vi "FTW-Inbox-Core-ConstructMessagePipe.vi"(5 "Actor Identity (empty to create unnamed actor)":string, 7 "Is Primary?":bool=TRUE, 11 "error in":errorcluster) -> (4 "Message Pipe":refnum<queue>, 6 "Resolved Actor Identity":string, 15 "error out":errorcluster)   [LabVIEW 2015]
uses:
  core/type/FTW-Type-JSON.ctl
panel:
  # "Inputs"
  # "Outputs"
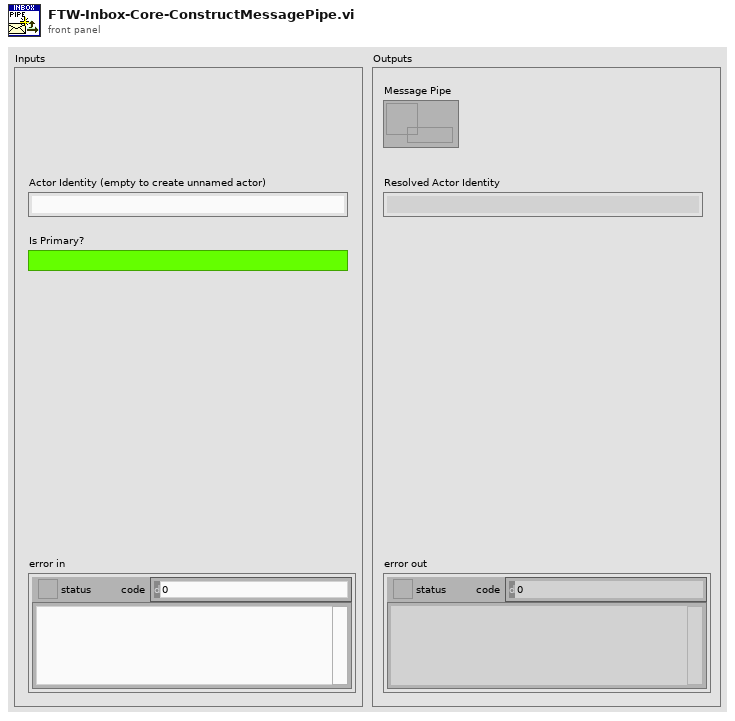
[diagram p1: front panel]
types:
  T1 = typedef "FTW-Type-JSON.ctl" = refnum<data-value>
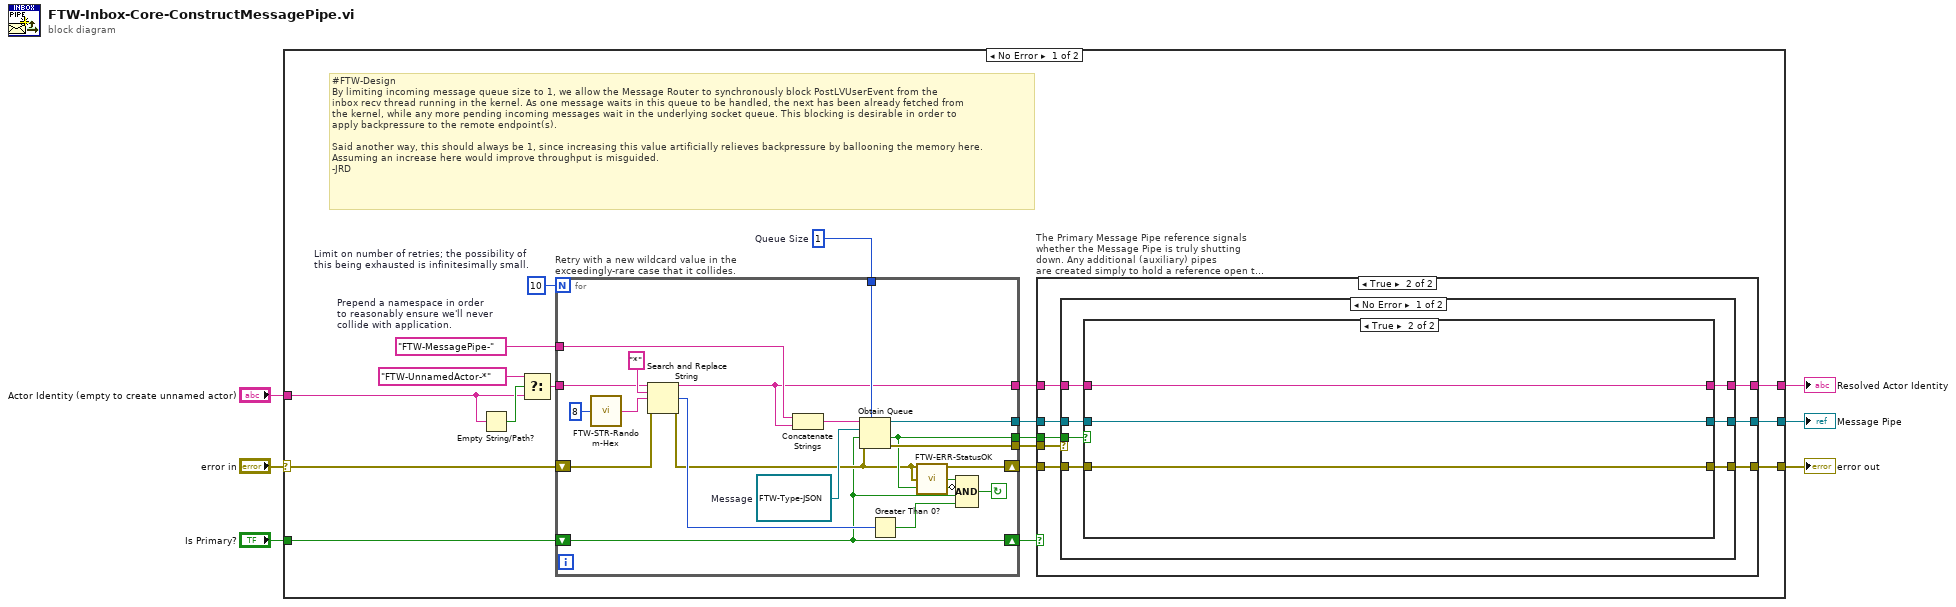
[diagram p0: block diagram]
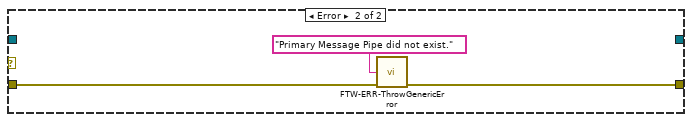
[diagram p3: hidden frame]
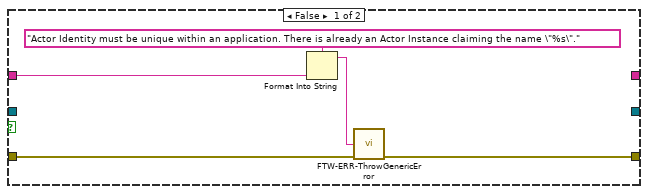
[diagram p4: hidden frame]
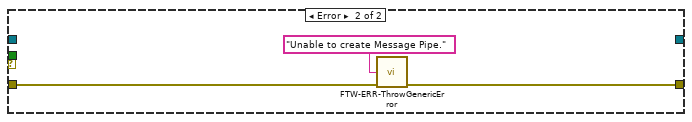
[diagram p5: hidden frame]
diagram:
  n1 = case shown="No Error" "error in" {
    selector: "error in" -> [w14 w83]
    tunnel: [w23 _] -> w6
    tunnel: "Actor Identity (empty to create unnamed actor)" -> [w16 _]
    tunnel: "Is Primary?" -> [w18 _]
    tunnel: [w24 w83] -> w3
    tunnel: [w19 _] -> w1
    frame No Error {
      w7 = "FTW-MessagePipe-"  # Prepend a namespace in order to reasonably ensure we'll never collide with application.
      w10 = 1  # Queue Size
      w11 = 10  # Limit on number of retries; the possibility of this being exhausted is infinitesimally small.
      # "#FTW-Design\nBy limiting incoming message queue size to 1, we allow the Message Router to synchronously block PostLVUserEvent from the\ninbox recv thread running in the kernel. As one message waits in this queue to be handled, the next has been already fetched from\nthe kernel, while any more pending incoming messages wait in the underlying socket queue. This blocking is desirable in order to\napply backpressure to the remote endpoint(s).\n\nSaid another way, this should always be 1, since increasing this value artificially relieves backpressure by ballooning the memory here.\nAssuming an increase here would improve throughput is misguided.\n-JRD"
      n2 = Empty String/Path?(string/path=w16) -> (empty?=w17:bool)
      n3 = Select(t="FTW-UnnamedActor-*" ("string"), s=w17, f=w16) -> (s? t:f=w8:string)
      n4 = for "Retry with a new wildcard value in the exceedingly-rare case that it collides." {
        N: w11 -> [_]
        tunnel: [w42] -> w21
        tunnel: [w41] -> w20
        shift-right: [w32] -> w13
        shift-left: w14 -> [w37]
        tunnel: [w33] -> w22
        tunnel: w8 -> [w34]
        tunnel: [w26] -> w12
        tunnel: w10 -> [w29]
        shift-right: [w28] -> w9
        shift-left: w18 -> [w28]
        tunnel: w7 -> [w27]
        stop <- w30 continue-if-true
        w43 = T1 refnum  # Message
        n5 = call "FTW-STR-Random-Hex.vi"("String Length"=8) -> ("Random Hex String"=w40:string)  [unwired: 3 in]
        n6 = Search and Replace String(input string=w34, search string="*", replace string=w40, error in=w37) -> (result string=w26:string, number of replacements=w36:i32, error out=w32:errorcluster)  [unwired: 4 in, 1 out]
        n7 = Concatenate Strings(w27, w26) -> (w25:string)
        n8 = Obtain Queue(max queue size (-1, unlimited)=w29, name (unnamed)=w25, element data type=w43, create if not found? (T)=w28, error in (no error)=w32) -> (queue out=w42:refnum<queue>, created new?=w33:bool, error out=w41:errorcluster)
        n9 = Greater Than 0?(x=w36) -> (x > 0?=w35:bool)
        n10 = call "FTW-ERR-StatusOK.vi"("error to check"=w32) -> ("Status OK?"=w31:bool)
        n11 = Compound Arithmetic op=AND(w31, invert w33, w28, w35) -> (w30:bool)
      }
      n12 = case "The Primary Message Pipe reference signals whether the Message Pipe is truly shutting down. Any additional (auxiliary) pipes\nare created simply to hold a reference open to existing messages in the pipe once it's shut down." shown="True" w9 {
        tunnel: w22 -> [_ w64]
        tunnel: w21 -> [w50 w63]
        tunnel: [w48 w62] -> w23
        tunnel: w20 -> [w47 w58]
        tunnel: [w49 w61] -> w24
        tunnel: w12 -> [w44 w60]
        tunnel: w13 -> [w46 w59]
        tunnel: [w45 w57] -> w19
        frame False {
          n13 = case shown="No Error" w47 {
            tunnel: w50 -> [w53 _]
            tunnel: [w52 w55] -> w49
            tunnel: [w53 _] -> w48
            tunnel: w46 -> [w52 w54]
            tunnel: [w51 _] -> w45
            tunnel: w44 -> [w51 _]
            frame No Error {
            }
            frame Error {
              n14 = call "FTW-ERR-ThrowGenericError.vi"("Error Message"="Primary Message Pipe did not exist.", "error in"=w54) -> ("error out"=w55:errorcluster)  [unwired: 13 in]
            }
          }
        }
        frame True {
          n15 = case shown="No Error" w58 {
            tunnel: w64 -> [w71 _]
            tunnel: w63 -> [w70 _]
            tunnel: [w69 _] -> w62
            tunnel: [w68 w80] -> w61
            tunnel: w60 -> [w67 _]
            tunnel: w59 -> [w66 w81]
            tunnel: [w65 _] -> w57
            frame No Error {
              n16 = case shown="True" w71 {
                tunnel: w70 -> [_ w79]
                tunnel: [_ w79] -> w69
                tunnel: w66 -> [w74 w78]
                tunnel: [w73 w78] -> w68
                tunnel: w67 -> [w72 w77]
                tunnel: [_ w77] -> w65
                frame False {
                  n17 = Format Into String(format string="Actor Identity must be unique within an application. There is already an Actor Instance claiming the name \"%s\"." ("Error Message"), w72) -> (resulting string=w75:string)  [unwired: 2 in, 1 out]
                  n18 = call "FTW-ERR-ThrowGenericError.vi"("Error Message"=w75, "error in"=w74) -> ("error out"=w73:errorcluster)  [unwired: 13 in]
                }
                frame True {
                }
              }
            }
            frame Error {
              n19 = call "FTW-ERR-ThrowGenericError.vi"("Error Message"="Unable to create Message Pipe.", "error in"=w81) -> ("error out"=w80:errorcluster)  [unwired: 13 in]
            }
          }
        }
      }
    }
    frame Error {
    }
  }
  "error out" <- w3
  "Message Pipe" <- w6
  "Resolved Actor Identity" <- w1
